vi "Add_tree.vi"(5 "Children Symbols":i32[][](array[numeric]), 7 "Parrent Symbol":i32[](array[numeric]), 8 "error in":errorcluster, 9 "Children":string[][](array[string]), 10 "Parent":string[](array[string]), 11 "Script_Tree":refnum<vi>) -> (0 "error IO":errorcluster, 3 "Script_Treeout":refnum<vi>)   [LabVIEW 2024, in "Setting_Screen.lvlib"]
uses:
  Setting_Screen.lvlib
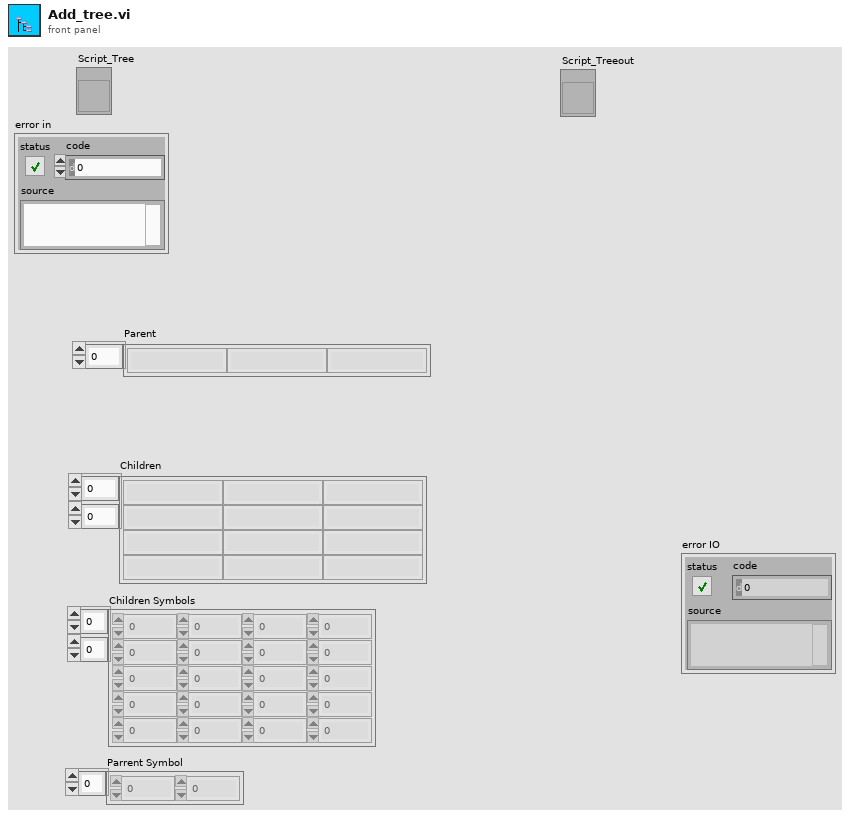
[diagram p1: front panel]
types:
  T1 = cluster{"Left Cell String":string, "Child Text":string[], "Child Tag":string, "Item Indent":i32, "Child Only?":bool, "Glyph Index":i32}[]
  T2 = cluster{"Left Cell String":string, "Child Text":string[], "Child Tag":string, "Item Indent":i32, "Child Only?":bool, "Glyph Index":i32}
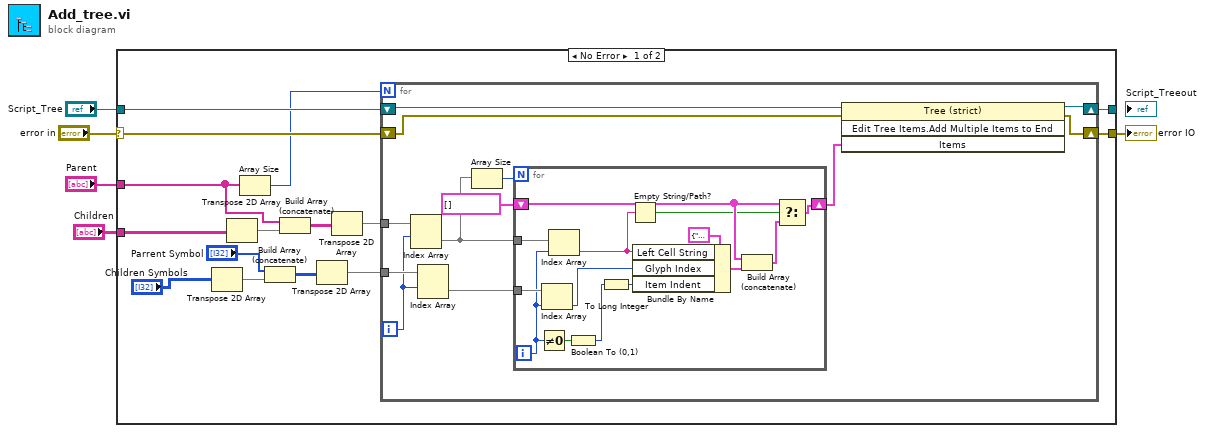
[diagram p0: block diagram]
diagram:
  n1 = case shown="No Error" "error in" {
    selector: "error in" -> [w20 w48]
    tunnel: "Parent" -> [w16 _]
    tunnel: "Script_Tree" -> [w19 w47]
    tunnel: "Children" -> [w17 _]
    tunnel: [w7 w47] -> _
    tunnel: [w6 w48] -> w1
    frame No Error {
      n2 = Transpose 2D Array(2D array="Children Symbols") -> (transposed array=w11:i32[][])
      n3 = Transpose 2D Array(2D array=w17) -> (transposed array=w15:string[][])
      n4 = Array Size(array=w16) -> (size(s)=w18:i32)
      n5 = Build Array (concatenate)("Parrent Symbol", w11) -> (w12:i32[][])
      n6 = Build Array (concatenate)(w16, w15) -> (w14:string[][])
      n7 = Transpose 2D Array(2D array=w12) -> (transposed array=w8:i32[][])
      n8 = Transpose 2D Array(2D array=w14) -> (transposed array=w13:string[][])
      n9 = for {
        N: w18 -> [_]
        shift-right: [w28] -> w6
        shift-left: w20 -> [w30]
        shift-right: [w29] -> w7
        shift-left: w19 -> [w31]
        tunnel: w13 -> [w32]
        tunnel: w8 -> [w27]
        i -> [w26]
        n10 = Index Array(array=w32, index (row)=w26) -> (element=w24:string[])  [unwired: 1 in]
        n11 = Index Array(array=w27, index (row)=w26) -> (element=w23:i32[])  [unwired: 1 in]
        n12 = Array Size(array=w24) -> (size(s)=w25:i32)
        n13 = for {
          N: w25 -> [_]
          tunnel: w24 -> [w46]
          tunnel: w23 -> [w45]
          shift-right: [w38] -> w21
          shift-left: T1 [] ("Items") -> [w42]
          i -> [w36]
          n14 = Not Equal To 0?(x=w36) -> (x != 0?=w35:bool)
          n15 = Index Array(array=w45, index=w36) -> (element=w37:i32)
          n16 = Index Array(array=w46, index=w36) -> (element=w41:string)
          n17 = Boolean To (0,1)(Boolean=w35) -> (0, 1=w34:i16)
          n18 = To Long Integer(number=w34) -> (32bit integer=w33:i32)
          n19 = Empty String/Path?(string/path=w41) -> (empty?=w40:bool)
          n20 = Bundle By Name(cluster=T2 {"Left Cell String"="", "Child Text"=[], "Child Tag"="", "Item Indent"=0, "Child Only?"=FALSE, "Glyph Index"=0} ("Item"), "Left Cell String"=w41, "Glyph Index"=w37, "Item Indent"=w33) -> (w43:T2)
          n21 = Build Array (concatenate)(w42, w43) -> (w39:T1)
          n22 = Select(t=w42, s=w40, f=w39) -> (s? t:f=w38:T1)
        }
        n23 = invoke class="Tree (strict)" method="Edit Tree Items.Add Multiple Items to End"(reference=w31, error in=w30, "Items"=w21) -> (reference out=w29:refnum<vi>, error out=w28:errorcluster)  [unwired: 1 in, 2 out]
      }
    }
    frame Error {
    }
  }
  "error IO" <- w1
